vi "My_RIGOL_v1_3_single_impulse.vi"() -> ()   [LabVIEW 2012]
panel:
  in  "Amplitude Unit (0: Vpp) 2":i32(ring) items=["Vpp", "Vrms", "dBm"]
  in  "Amplitude Диода (5 Vpp) 2":dbl=5.0
  in  "Amplitude Unit (0: Vpp)":i32(ring) items=["Vpp", "Vrms", "dBm"]
  in  "Amplitude Детектора (5 Vpp)":dbl=5.0
  in  "VISA":refnum<visa-resource-name>
  out "Сигнал Детектора":cluster{"Y":dbl[], "Y":dbl[]}[](graph) caption="XY Graph 3"
  out "Сигнал Диода":cluster{"Y":dbl[], "Y":dbl[]}[](graph) caption="XY Graph 3"
  out "Разница между \nсигналом диода и детектора, с":dbl format="%.12p"
  in  "Сколько точек\n сдвигать":i32
  out "Начало интервала":string
  out "Оставшиеся точки":string
  out "Начало второго импульса":string
  out "Количество точек":string caption="String"
  in  "Время между импульсами, с 2":dbl format="%#_12p"
  in  "Ширина импульса, с 2":dbl=1000.0 format="%#_12p"
  out "Начало интервала":string
  out "Оставшиеся точки":string caption="String 3"
  out "Начало второго импульса":string
  out "Количество точек":string caption="String"
  in  "Количество точек":dbl
  in  "Время между импульсами, с":dbl format="%#_12p"
  in  "Ширина импульса, с":dbl=1000.0 format="%#_12p"
  out "Выход на канал 2":string
  out "Выход на канал 1":string
  in  "Частота (1000 Hz)":dbl=1000.0 format="%#_12p"
  # "Chanel 2"
  # "Chanel 1"
  # "ДИОД"
  # "ДЕТЕКТОР"
  # "ДЕТЕКТОР"
  # "ДИОД"
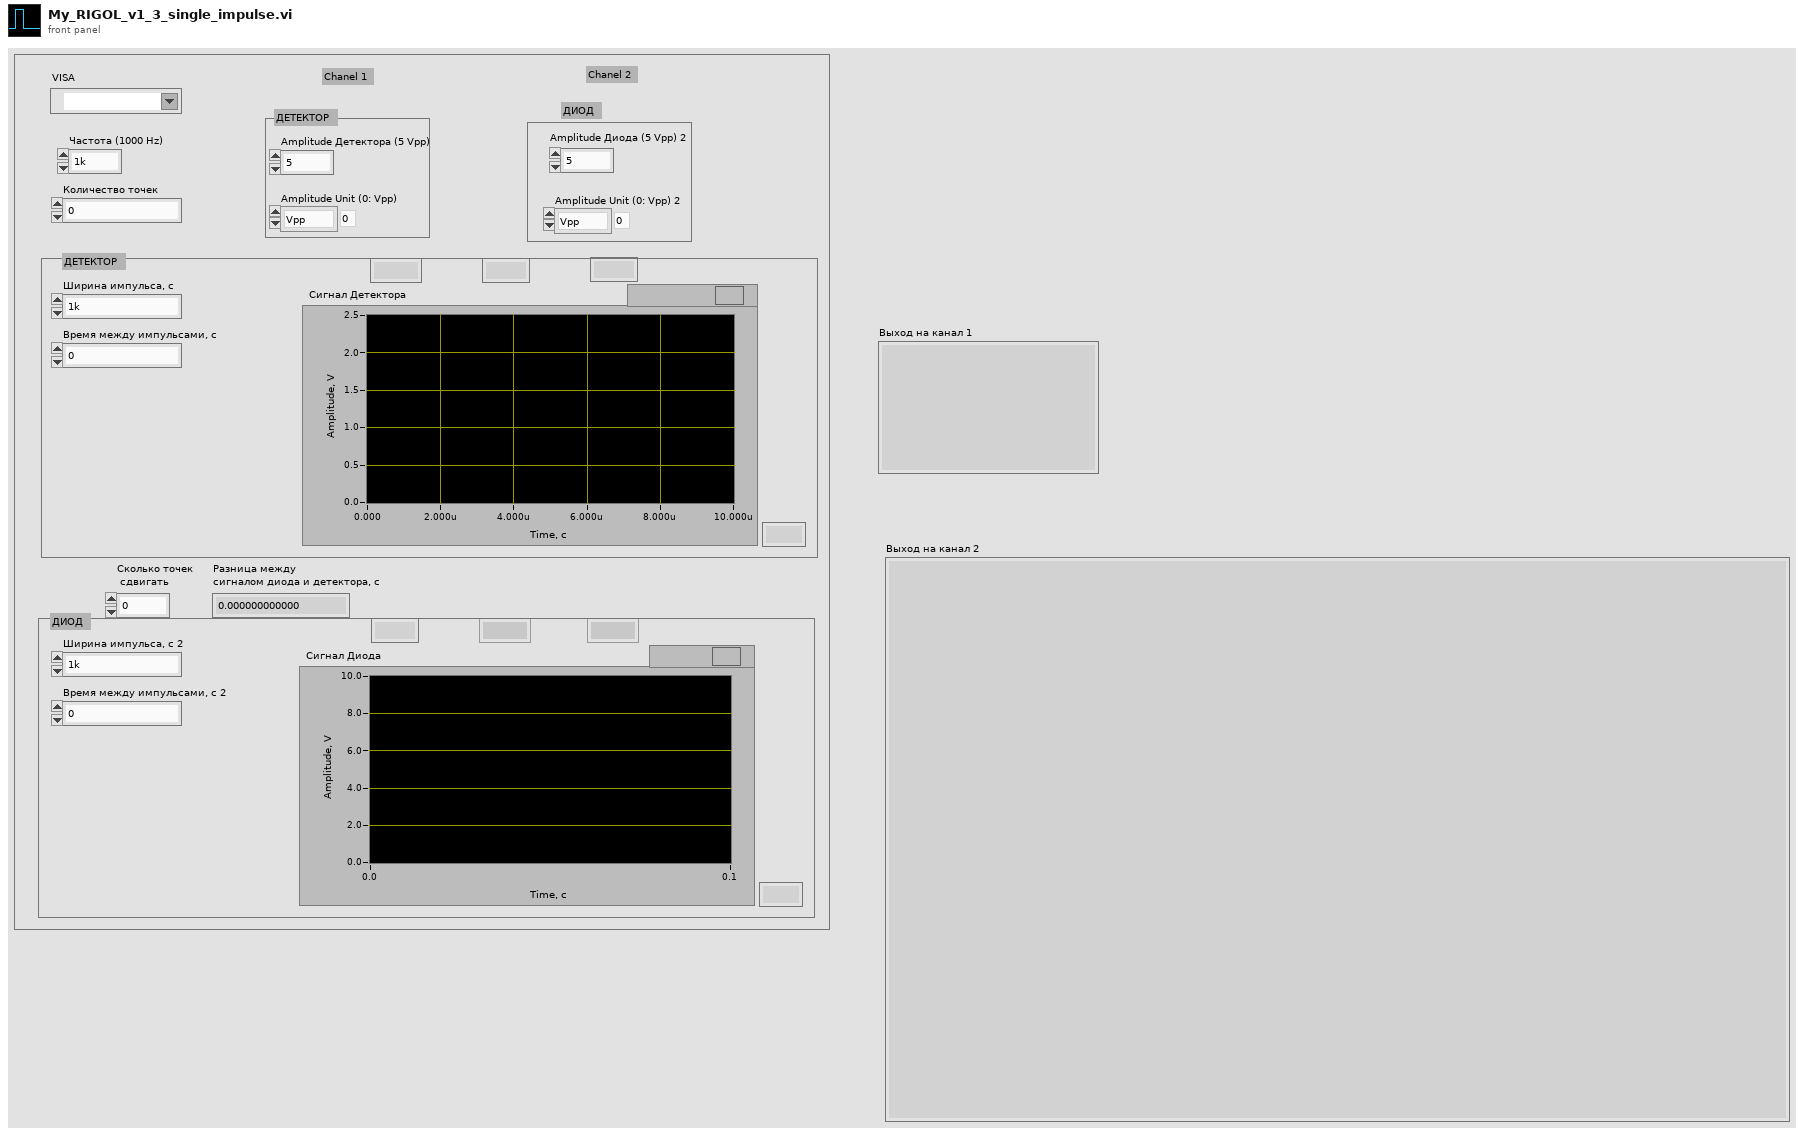
[diagram p1: front panel]
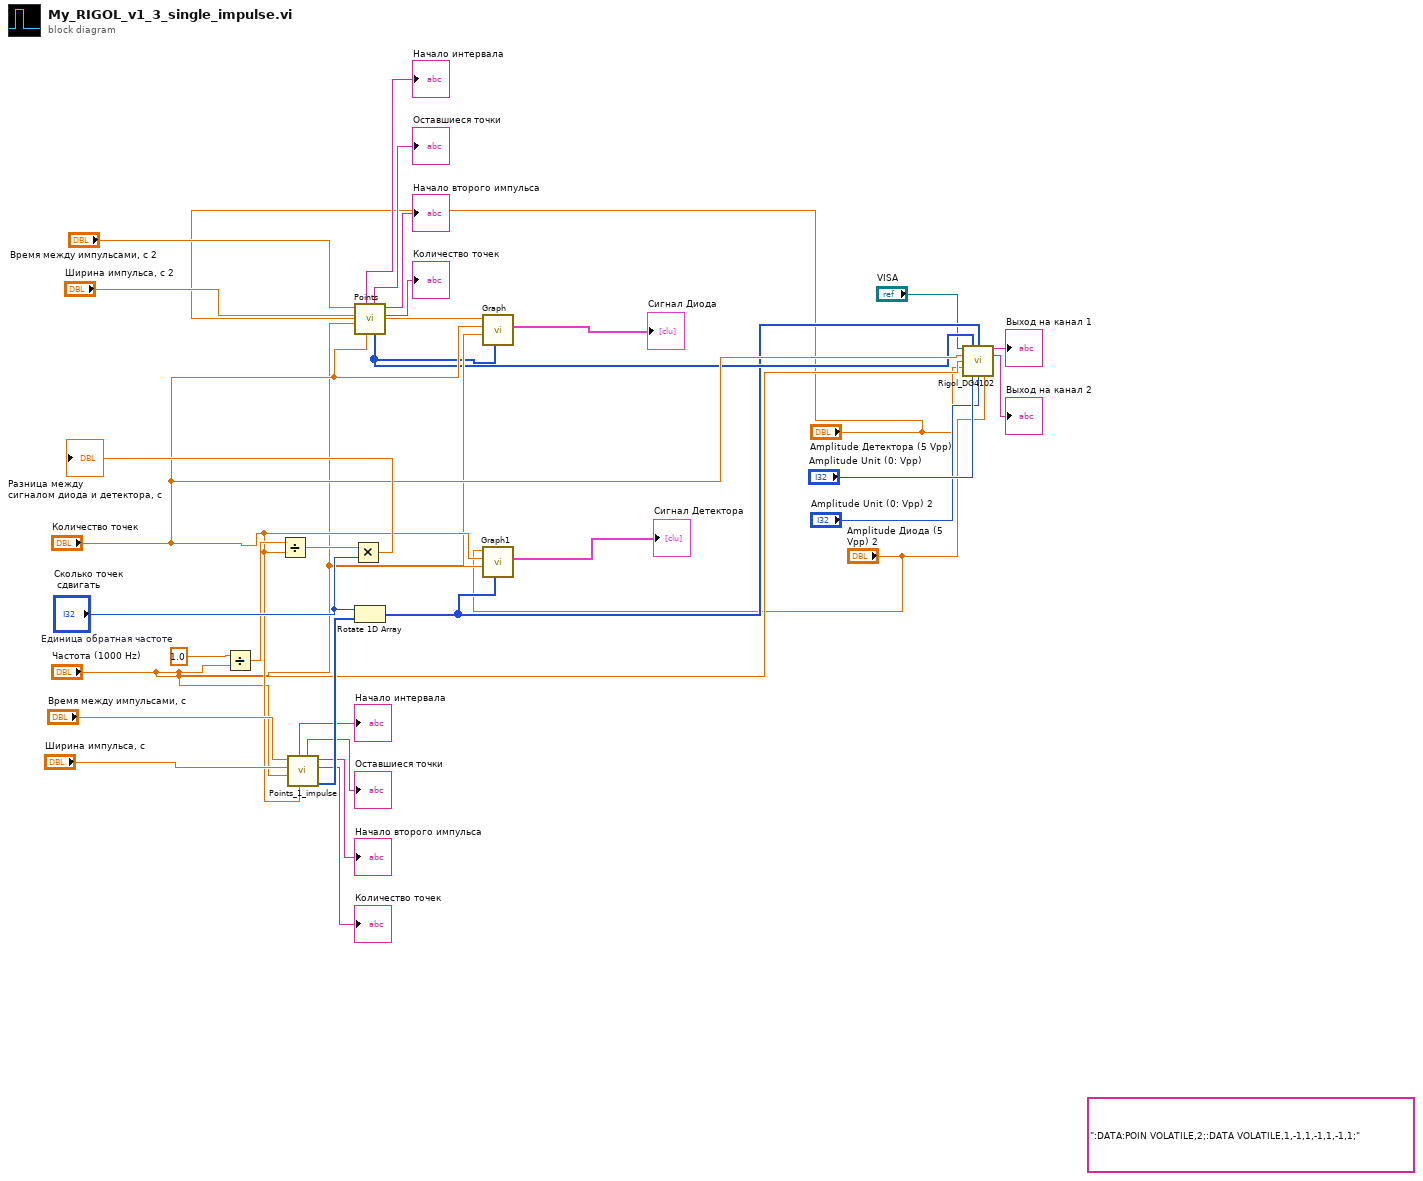
[diagram p0: block diagram]
diagram:
  w14 = 1.0  # Единица обратная частоте
  (unwired) ":DATA:POIN VOLATILE,2;:DATA VOLATILE,1,-1,1,-1,1,-1,1;"
  n1 = Divide(x=w14, y="Частота (1000 Hz)") -> (x/y=w15:dbl)
  n2 = Divide(x=w15, y="Количество точек") -> (x/y=w13:dbl)
  n3 = call "Points_1_impulse.vi"("Количество точек"="Количество точек", "Частота (1000 Hz)"="Частота (1000 Hz)", "Ширина импульса, с"="Ширина импульса, с", "Время между импульсами, с"="Время между импульсами, с") -> ("Детектор"=w23:i32[], "Количество точек"=→"Количество точек":string, "Начало второго импульса"=→"Начало второго импульса":string, "Оставшиеся точки"=→"Оставшиеся точки":string, "Начало интервала"=→"Начало интервала":string)  [unwired: 2 in, 1 out]
  n4 = Multiply(x=w13, y="Сколько точек\n сдвигать") -> (x*y=→"Разница между \nсигналом диода и детектора, с":dbl)
  n5 = call "Points.vi"("Количество точек"="Количество точек", "Частота (1000 Hz)"="Частота (1000 Hz)", "Ширина импульса, с"="Ширина импульса, с 2", "Время между импульсами, с"="Время между импульсами, с 2") -> ("Количество точек"=→"Количество точек":string, "Начало второго импульса"=→"Начало второго импульса":string, "Диод"=w7:i32[], "Оставшиеся точки"=→"Оставшиеся точки":string, "Начало интервала"=→"Начало интервала":string)  [unwired: 2 in, 1 out]
  n6 = Rotate 1D Array(1:w23, 2:"Сколько точек\n сдвигать") -> (0:w6:i32[])
  n7 = call "Graph.vi"("Array"=w7, "Частота (1000 Hz)"="Частота (1000 Hz)", "Количество точек"="Количество точек", "Амплитуда"="Amplitude Детектора (5 Vpp)") -> ("XY Graph 3"=→"Сигнал Диода":cluster{"Y":dbl[], "Y":dbl[]}[])  [unwired: 7 in]
  n8 = call "Graph1.vi"("Массив точек"=w6, "Частота (1000 Hz)"="Частота (1000 Hz)", "Количество точек"="Количество точек", "Амплитуда оси Y"="Amplitude Диода (5 Vpp) 2") -> ("График"=→"Сигнал Детектора":cluster{"Y":dbl[], "Y":dbl[]}[])  [unwired: 7 in]
  n9 = call "Rigol_DG4102.vi"("VISA Refnum in"="VISA", "Массив диода"=w7, "Масиив детектора"=w6, "Количество точек"="Количество точек", "Частота (1000 Hz)"="Частота (1000 Hz)", "Amplitude (5 Vpp)"="Amplitude Детектора (5 Vpp)", "Amplitude Unit (0: Vpp)"="Amplitude Unit (0: Vpp)", "Amplitude Unit (0: Vpp) 2"="Amplitude Unit (0: Vpp) 2", "Amplitude (5 Vpp) 2"="Amplitude Диода (5 Vpp) 2") -> ("Выход на канал 1"=→"Выход на канал 1":string, "Выход на канал 2"=→"Выход на канал 2":string)  [unwired: 5 in]
